vi "example_tcp.vi"() -> ()   [LabVIEW 2017, in "libirimager_direct_binding.lvlib"]
uses:
  libirimager_direct_binding.lvlib
panel:
  out "Thermal Image":picture
  out "function return savepng":i32
  in  "triggerFlag":bool
  out "function return triggerAutoflag":i32
  in  "set_trigger_mode":bool
  in  "state":i32
  out "function return setAutoflag":i32
  in  "terminate":bool
  out "function return terminate":i32
  in  "getThm":bool
  out "function return thm":i32
  out "thermal data out":u16[](array[numeric])
  in  "connect_tcp":bool
  in  "ip":string="localhost"
  in  "port":i32=1337
  out "function return":i32
  out "w out":i32
  out "h out":i32
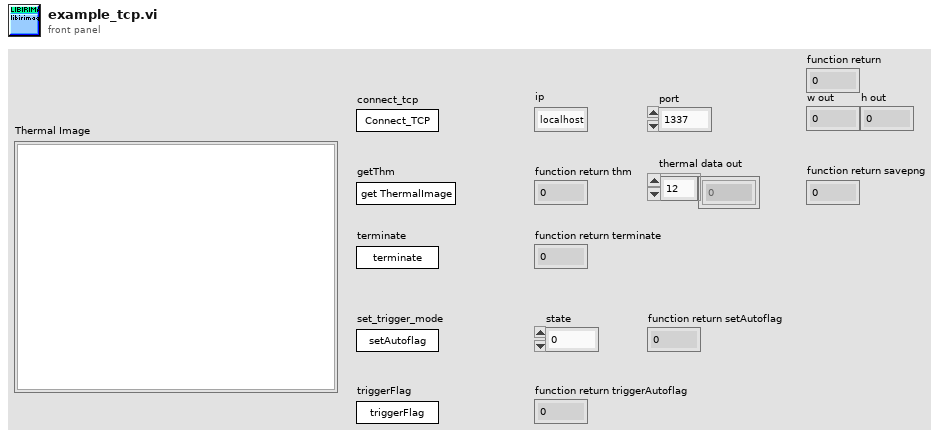
[diagram p1: front panel]
types:
  T1 = typedef "imagedata.ctl" = cluster{"image type":i32, "image depth":i32, "image":u8[], "mask":u8[], "colors":u32[], "Rectangle":cluster{"left":i16, "top":i16, "right":i16, "bottom":i16}}
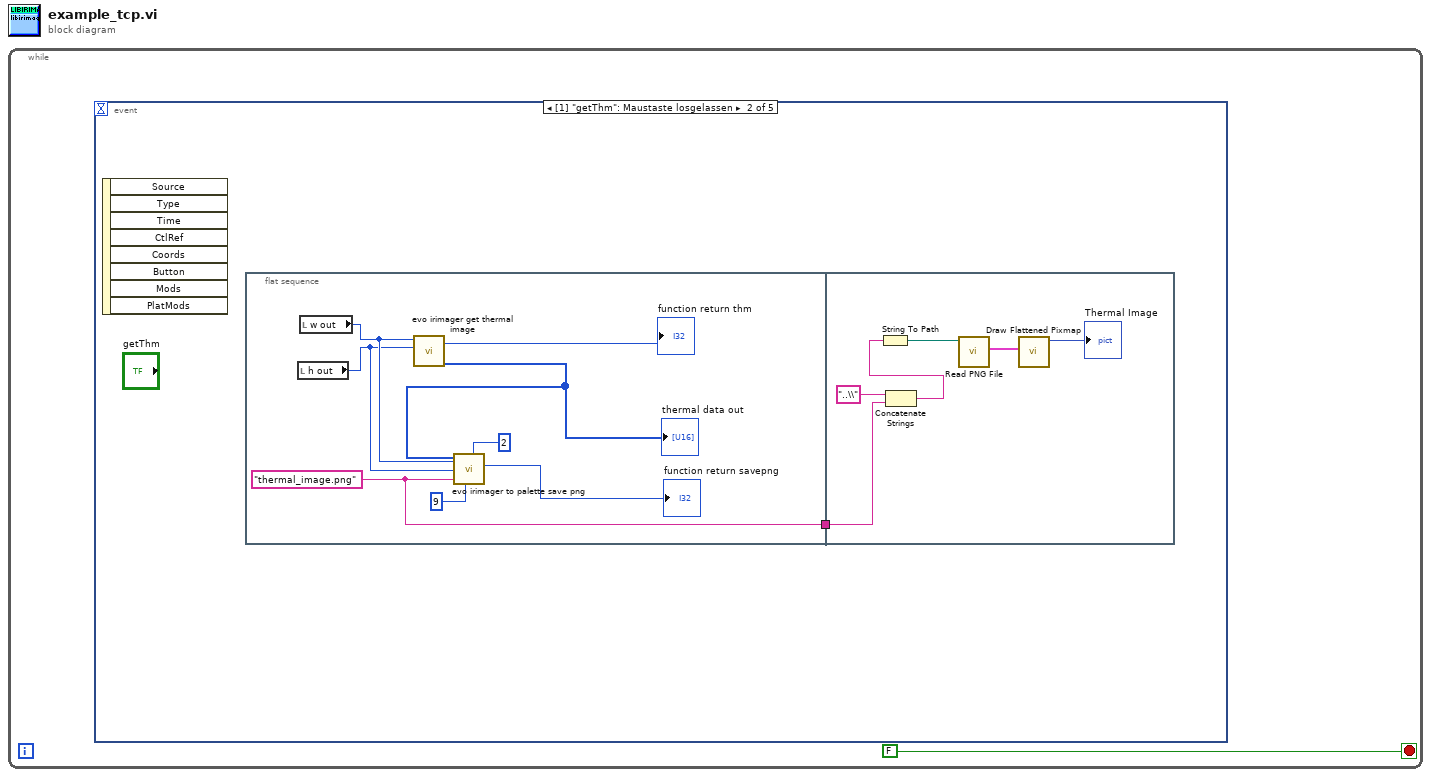
[diagram p0: block diagram]
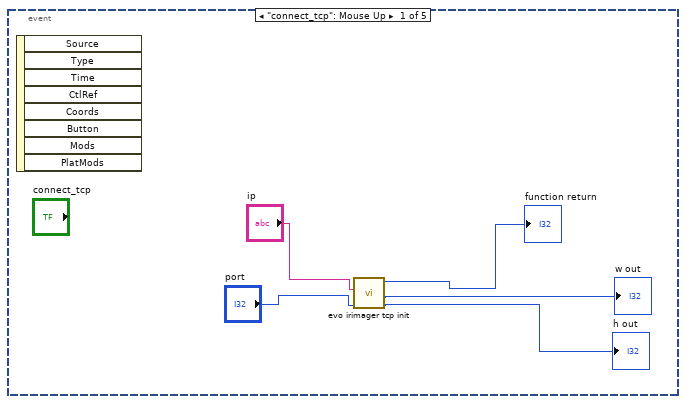
[diagram p2: hidden frame]
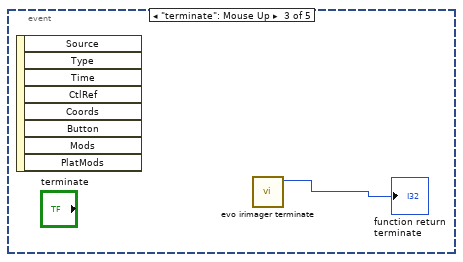
[diagram p3: hidden frame]
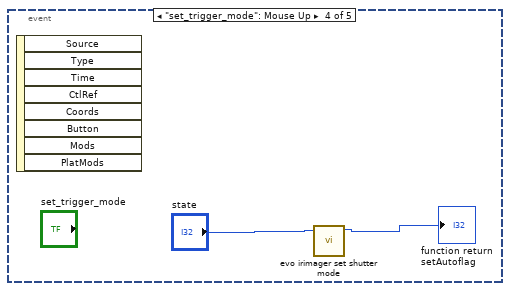
[diagram p4: hidden frame]
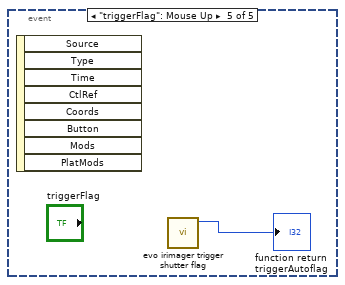
[diagram p5: hidden frame]
diagram:
  n1 = while {
    stop <- FALSE stop-if-true
    n2 = event shown="[1] \"getThm\": Maustaste losgelassen" {
      selector: _ -> [_ _ _ _ _]
      dyn-events: _ -> [_ _ _ _ _]
      timeout: _ -> [_ _ _ _ _]
      event "connect_tcp": Mouse Up {
        n3 = event-data() -> ()  [unwired: 1 in, 8 out]
        n4 = call "evo irimager tcp init.vi"("port"="port", "ip"="ip") -> ("h out"=→"h out":i32, "w out"=→"w out":i32, "function return 2"=→"function return":i32)  [unwired: 7 in]
      }
      event "getThm": Mouse Up {
        n5 = event-data() -> ()  [unwired: 1 in, 8 out]
        n6 = flat-sequence {
          tunnel: [w8] -> w7
          tunnel: w7 -> [w17]
          frame #0 {
            w8 = "thermal_image.png" ("path")
            n7 = local read "h out"() -> (w12:i32)
            n8 = local read "w out"() -> (w13:i32)
            n9 = call "evo irimager get thermal image.vi"("h"=w12, "w"=w13) -> ("data out"=w14:u16[], "function return"=→"function return thm":i32)  [unwired: 6 in, 2 out]
            "thermal data out" <- w14
            n10 = call "evo irimager to palette save png.vi"("palette_scale"=2, "palette"=9, "path"=w8, "h"=w12, "w"=w13, "thermal_data"=w14) -> ("function return"=→"function return savepng":i32)  [unwired: 4 in, 1 out]
          }
          frame #1 {
            n11 = Concatenate Strings("..\\" ("String"), w17) -> (w18:string)
            n12 = String To Path(string=w18) -> (path=w19:path)
            n13 = call <vilib>:"Read PNG File.vi"("path to PNG file"=w19) -> ("image data"=w20:T1)  [unwired: 8 in, 2 out]
            n14 = call <vilib>:"Draw Flattened Pixmap.vi"("image data"=w20) -> ("new picture"=→"Thermal Image":picture)  [unwired: 8 in]
          }
        }
      }
      event "terminate": Mouse Up {
        n15 = event-data() -> ()  [unwired: 1 in, 8 out]
        n16 = call "evo irimager terminate.vi"() -> ("function return"=→"function return terminate":i32)  [unwired: 11 in]
      }
      event "set_trigger_mode": Mouse Up {
        n17 = event-data() -> ()  [unwired: 1 in, 8 out]
        n18 = call "evo irimager set shutter mode.vi"("mode"="state") -> ("function return"=→"function return setAutoflag":i32)  [unwired: 10 in]
      }
      event "triggerFlag": Mouse Up {
        n19 = event-data() -> ()  [unwired: 1 in, 8 out]
        n20 = call "evo irimager trigger shutter flag.vi"() -> ("function return"=→"function return triggerAutoflag":i32)  [unwired: 11 in]
      }
    }
  }
